vi "parse and check websocket headers.vi"(7 "accept key":string, 8 "error in":errorcluster, 9 "timeout ms":i32, 10 "max header size":i32, 11 "TCP Network Connection in":refnum<k5>) -> (0 "error out":errorcluster, 3 "headers":T1)   [LabVIEW 2016, in "websocket client.lvclass"]
uses:
  websocket client.lvclass
  HTTP server/http header data.ctl
  <vilib>/dlg_ctls.llb/Space Constant.vi
  HTTP server/headers/http headers.lvlib
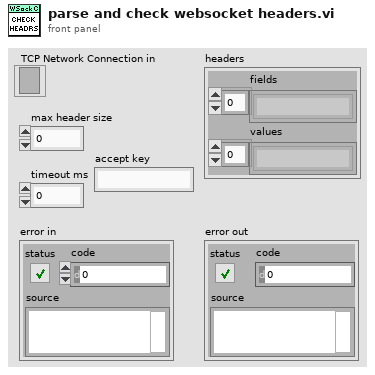
[diagram p1: front panel]
types:
  T1 = typedef "http headers.lvlib/http header data.ctl" = cluster{"fields":string[], "values":string[]}
  T2 = enum16{"Standard", "Buffered", "CRLF", "Immediate"}
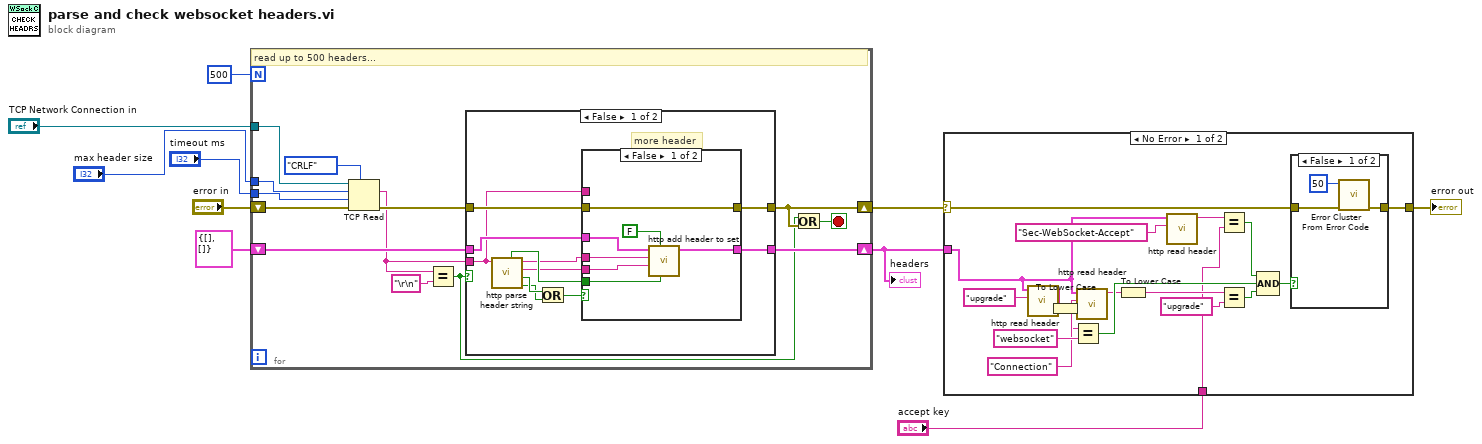
[diagram p0: block diagram]
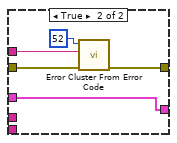
[diagram p4: hidden frame]
diagram:
  n1 = for {
    N: 500 -> [_]
    tunnel: "TCP Network Connection in" -> [w22]
    tunnel: "max header size" -> [w21]
    tunnel: "timeout ms" -> [w20]
    shift-right: [w14] -> w8
    shift-left: "error in" -> [w19]
    shift-right: [w17] -> w10
    shift-left: T1 {"fields"=[], "values"=[]} ("headers") -> [w18]
    stop <- w12 stop-if-true
    # "read up to 500 headers..."
    n2 = TCP Read(connection ID=w22, bytes to read=w21, error in (no error)=w19, 7:T2."CRLF" ("mode (standard)"), 9:w20) -> (data out=w15:string, error out=w16:errorcluster)  [unwired: 1 out]
    n3 = Equal?(x=w15, y="\r\n" ("x")) -> (x = y?=w11:bool)
    n4 = case shown="False" w11 {
      tunnel: w18 -> [w34 w47]
      tunnel: [w33 w47] -> w17
      tunnel: w16 -> [w29 w48]
      tunnel: w15 -> [w24 _]
      tunnel: [w25 w48] -> w14
      frame False {
        # "more header"
        n5 = call "http parse header string.vi"("raw string"=w24) -> ("no field name"=w26:bool, "no crlf"=w28:bool, "header field data"=w30:string, "header field name"=w31:string, "continuation"=w32:bool)  [unwired: 6 in]
        n6 = Or(x=w28, y=w26) -> (x .or. y?=w27:bool)
        n7 = case shown="False" w27 {
          tunnel: w34 -> [w41 w44]
          tunnel: [w40 w44] -> w33
          tunnel: w32 -> [w38 _]
          tunnel: w31 -> [w37 _]
          tunnel: w30 -> [w36 _]
          tunnel: [w35 w45] -> w25
          tunnel: w29 -> [w35 w46]
          tunnel: w24 -> [_ w42]
          frame False {
            n8 = call "http add header to set.vi"("continuation?"=w38, "override on duplicate?"=FALSE, "header field data"=w36, "header field name"=w37, "headers in"=w41) -> ("headers out"=w40:T1)  [unwired: 6 in]
          }
          frame True {
            n9 = call <vilib>:"Error Cluster From Error Code.vi"("error in (no error)"=w46, "error message (\"\")"=w42, "error code (0)"=52) -> ("error out"=w45:errorcluster)  [unwired: 6 in]
          }
        }
      }
      frame True {
        # "clrf before body (which should be empty)"
      }
    }
    n10 = Or(x=w11, y=w14) -> (x .or. y?=w12:bool)
  }
  "headers" <- w10
  n11 = case shown="No Error" w8 {
    selector: w8 -> [w51 w71]
    tunnel: w10 -> [w66 _]
    tunnel: [w52 w71] -> w9
    tunnel: "accept key" -> [w50 _]
    frame No Error {
      n12 = call "http read header.vi"("header field name"="upgrade", "headers"=w66) -> ("value"=w63:string)  [unwired: 8 in, 1 out]
      n13 = To Lower Case(string=w63) -> (all lower case string=w49:string)
      n14 = Equal?(x=w49, y="websocket") -> (x = y?=w59:bool)
      n15 = call "http read header.vi"("header field name"="Connection", "headers"=w66) -> ("value"=w57:string)  [unwired: 8 in, 1 out]
      n16 = To Lower Case(string=w57) -> (all lower case string=w56:string)
      n17 = call "http read header.vi"("header field name"="Sec-WebSocket-Accept", "headers"=w66) -> ("value"=w64:string)  [unwired: 8 in, 1 out]
      n18 = Equal?(x=w64, y=w50) -> (x = y?=w60:bool)
      n19 = Equal?(x=w56, y="upgrade") -> (x = y?=w54:bool)
      n20 = Compound Arithmetic op=AND(w60, w59, w54) -> (w53:bool)
      n21 = case shown="False" w53 {
        tunnel: [w68 w70] -> w52
        tunnel: w51 -> [w69 w70]
        frame False {
          n22 = call <vilib>:"Error Cluster From Error Code.vi"("error in (no error)"=w69, "error code (0)"=50) -> ("error out"=w68:errorcluster)  [unwired: 7 in]
        }
        frame True {
        }
      }
    }
    frame Error {
    }
  }
  "error out" <- w9
